vi "Close.vi"(8 "error in (no error)":errorcluster, 11 "PwrMtr_RSNRPZ in":refnum<class "PwrMtr_RSNRPZ.lvclass">) -> (0 "error out":errorcluster)   [LabVIEW 2014, in "PwrMtr_RSNRPZ.lvclass"]
uses:
  PwrMtr_RSNRPZ.lvclass
  PwrMtr_RSNRPZ.lvclass/PwrMtr_RSNRPZ.ctl
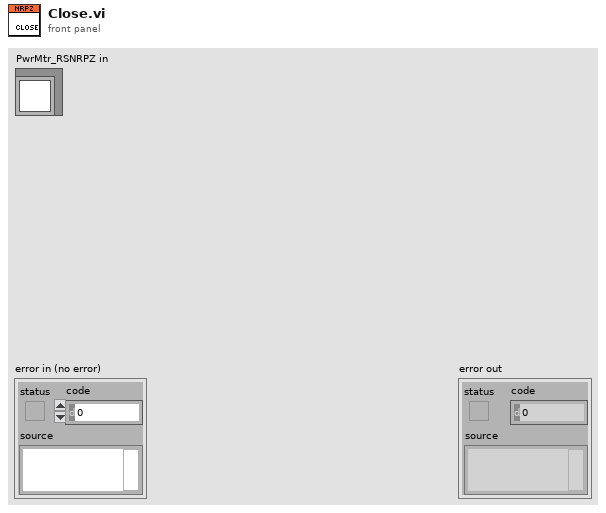
[diagram p1: front panel]
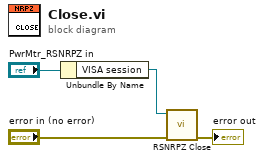
[diagram p0: block diagram]
diagram:
  n1 = Unbundle By Name("PwrMtr_RSNRPZ in") -> ("VISA session"=w1:refnum<visa-resource-name>)
  n2 = call <instrlib>:"RSNRPZ Close.vi"("error in (no error)"="error in (no error)", "VISA session"=w1) -> ("error out"=→"error out":errorcluster)  [unwired: 9 in]
